vi "PRBS Test.vi"() -> ()   [LabVIEW 2015]
uses:
  PRBScontrol.ctl
panel:
  out "Finalizado?":bool
  out "PRBS out":u8[](array[numeric])
  out "error out":errorcluster
  in  "Action":T1
  in  "Periodo":i32
  in  "Duração da excitação (s)":i32
  in  "Seed bomba 1":i32
  in  "Seed bomba 2":i32
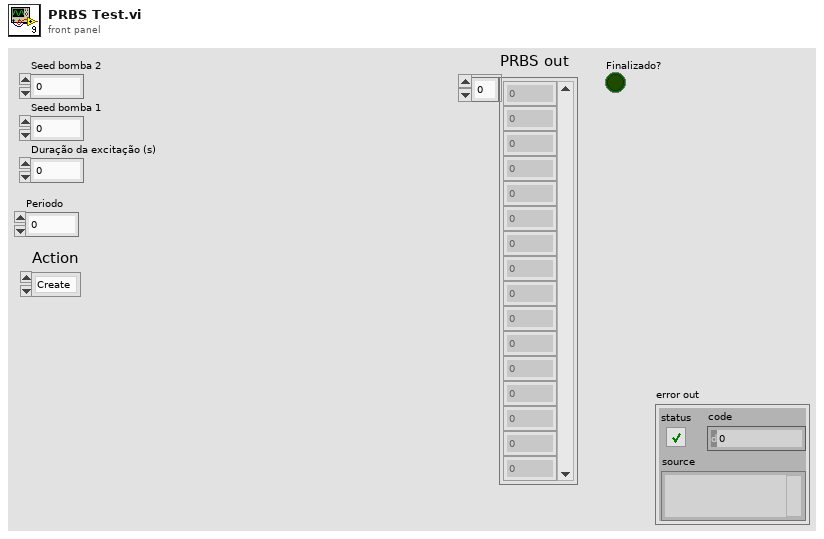
[diagram p1: front panel]
types:
  T1 = typedef "PRBScontrol.ctl" = enum16{"Create", "Get data point"}
  T2 = cluster{"seed":i64, "samples":i64, "upsampling factor":i32, "polynomial order":i32}[]
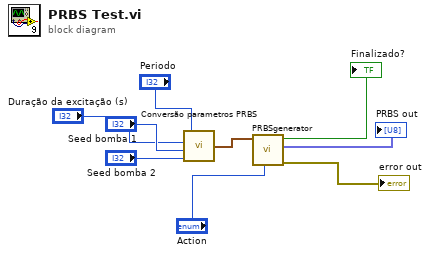
[diagram p0: block diagram]
diagram:
  n1 = call "Conversão parametros PRBS.vi"("Seed bomba 2"="Seed bomba 2", "Seed bomba 1"="Seed bomba 1", "Duração da excitação (s)"="Duração da excitação (s)", "Periodo"="Periodo") -> ("PRBS Parameters"=w9:T2)
  n2 = call "PRBSgenerator.vi"("Action"="Action", "PRBS Parameters"=w9) -> ("error out"=→"error out":errorcluster, "PRBS out"=→"PRBS out":fxp<+/-,20,5>[], "Finalizado?"=→"Finalizado?":bool)  [unwired: 7 in]
